vi "n64_generate_grid.vi"(8 "Tare":bool=TRUE, 9 "Row Length":i32=64, 10 "No. Nodes":i32=64, 11 "Sensor Readings (PACKET)":i16[](array[numeric])) -> (0 "Node XYZ List":dbl[][](array[numeric]), 1 "Y (GRID)":dbl[][](array[numeric]), 2 "X (GRID)":dbl[][](array[numeric]), 3 "Z (GRID)":dbl[][](array[numeric]))   [LabVIEW 2016]
uses:
  <vilib>/Math Plots/3D Math Plots/3D Quiver/3D Quiver XCtrl/3D Quiver.xctl
  <vilib>/Math Plots/3D Math Plots/3D Quiver/3D Quiver Datatype/Public/Plot Helper (Matrix).vi
  <vilib>/Math Plots/3D Math Plots/3D Quiver/3D Quiver Datatype/3D Quiver Datatype.lvclass
panel:
  in  "Tab Control":enum32{"16 Node", "64 Node"}(tab)
  in  "Lookup Index n16":i32[](array[numeric])=[0, 1, 2, 3, 4, 5, 6, 7, 8, 9, 10, 11, 12, 13, 14, 15]
  in  "Inv Gain n16":i32[][](array[numeric])=[[1, 1, 1], [1, 1, 1], [1, 1, 1], [1, 1, 1], [1, 1, 1], [1, 1, 1], [1, 1, 1], [1, 1, 1], [1, 1, 1], [1, 1, 1], [1, 1, 1], [1, 1, 1], [1, 1, 1], [1, 1, 1], [1, 1, 1], [1, 1, 1]]
  in  "Lookup Index n64":i32[](array[numeric])=[0, 1, 2, 3, 4, 5, 6, 7, 8, 9, 10, 11, 12, 13, 14, 15, 16, 17, 18, 19, 20, 21, 22, 23, 24, 25, 26, 27, 28, 29, 30, 31, 32, 33, 34, 35, 36, 37, 38, 39, 40, 41, 42, 43, 44, 45, 46, 47, 48, 49, 50, 51, 52, 53, 54, 55, 56, 57, 58, 59, 60, 61, 62, 63]
  in  "Inv Gain n64":i32[][](array[numeric])=[[1, 1, 1], [1, 1, 1], [1, 1, 1], [1, 1, 1], [1, 1, 1], [1, 1, 1], [1, 1, 1], [1, 1, 1], [1, 1, 1], [1, 1, 1], [1, 1, 1], [1, 1, 1], [1, 1, 1], [1, 1, 1], [1, 1, 1], [1, 1, 1], [1, 1, 1], [1, 1, 1], [1, 1, 1], [1, 1, 1], [1, 1, 1], [1, 1, 1], [1, 1, 1], [1, 1, 1], [1, 1, 1], [1, 1, 1], [1, 1, 1], [1, 1, 1], [1, 1, 1], [1, 1, 1], [1, 1, 1], [1, 1, 1], [1, 1, 1], [1, 1, 1], [1, 1, 1], [1, 1, 1], [1, 1, 1], [1, 1, 1], [1, 1, 1], [1, 1, 1], [1, 1, 1], [1, 1, 1], [1, 1, 1], [1, 1, 1], [1, 1, 1], [1, 1, 1], [1, 1, 1], [1, 1, 1], [1, 1, 1], [1, 1, 1], [1, 1, 1], [1, 1, 1], [1, 1, 1], [1, 1, 1], [1, 1, 1], [1, 1, 1], [1, 1, 1], [1, 1, 1], [1, 1, 1], [1, 1, 1], [1, 1, 1], [1, 1, 1], [1, 1, 1], [1, 1, 1]]
  in  "Tare":dbl[][](array[numeric])=[[0.00018775, -0.000174232, 3312.98], [0.000139686, -0.00039953199999999997, 2906.42], [-0.000288384, -0.001229387, 2606.34], [-3.6799e-05, -0.0012016, 3702.6], [0.000266605, -0.001108476, 3847.7999999999997], [0.00038301, -0.000208027, 3472.7], [-0.000177236, -0.000316171, 3651.7799999999997], [-0.00024557699999999997, 0.000544475, 4767.4], [-5.6325e-05, -0.00041305, 4172.08], [8.4112e-05, 0.000956774, 2562.7799999999997], [-0.000261348, 0.001097962, 3675.98], [-0.00014944899999999998, -0.00066839, 4856.94], [-0.000204272, 0.000920726, 4740.78], [-0.000242573, -7.7353e-05, 4009.94], [0.000246328, -0.000138184, 4358.42], [7.51e-06, 0.000451351, 5829.78]]
  out "3D Quiver":refnum<class "3D Plot Datatype.lvclass">[](xcontrol)
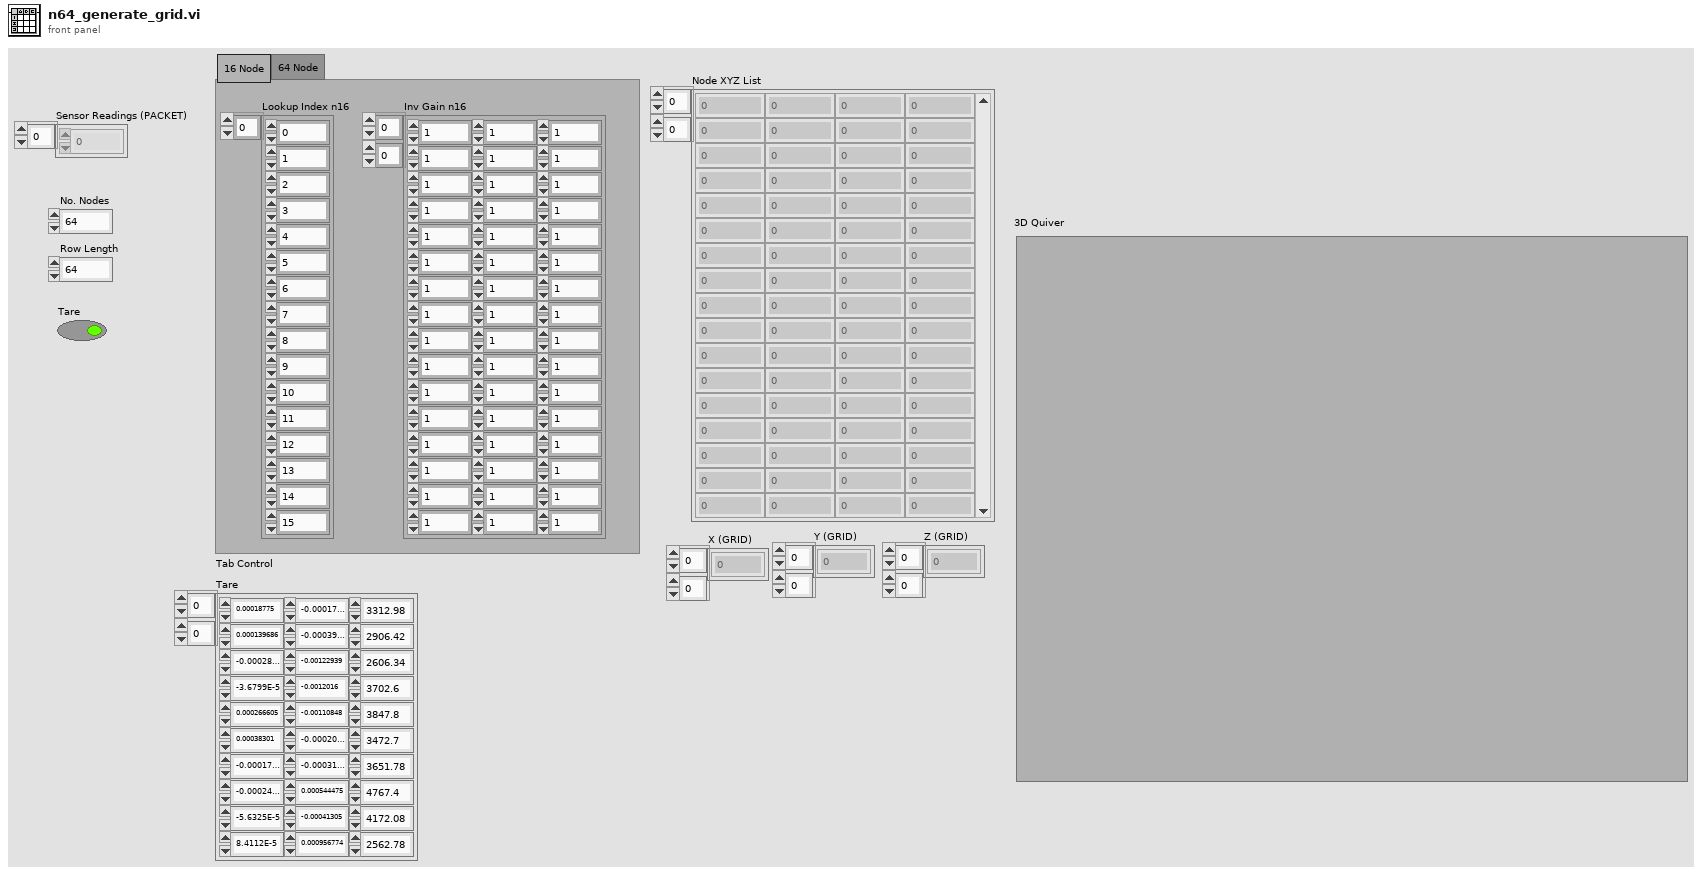
[diagram p1: front panel]
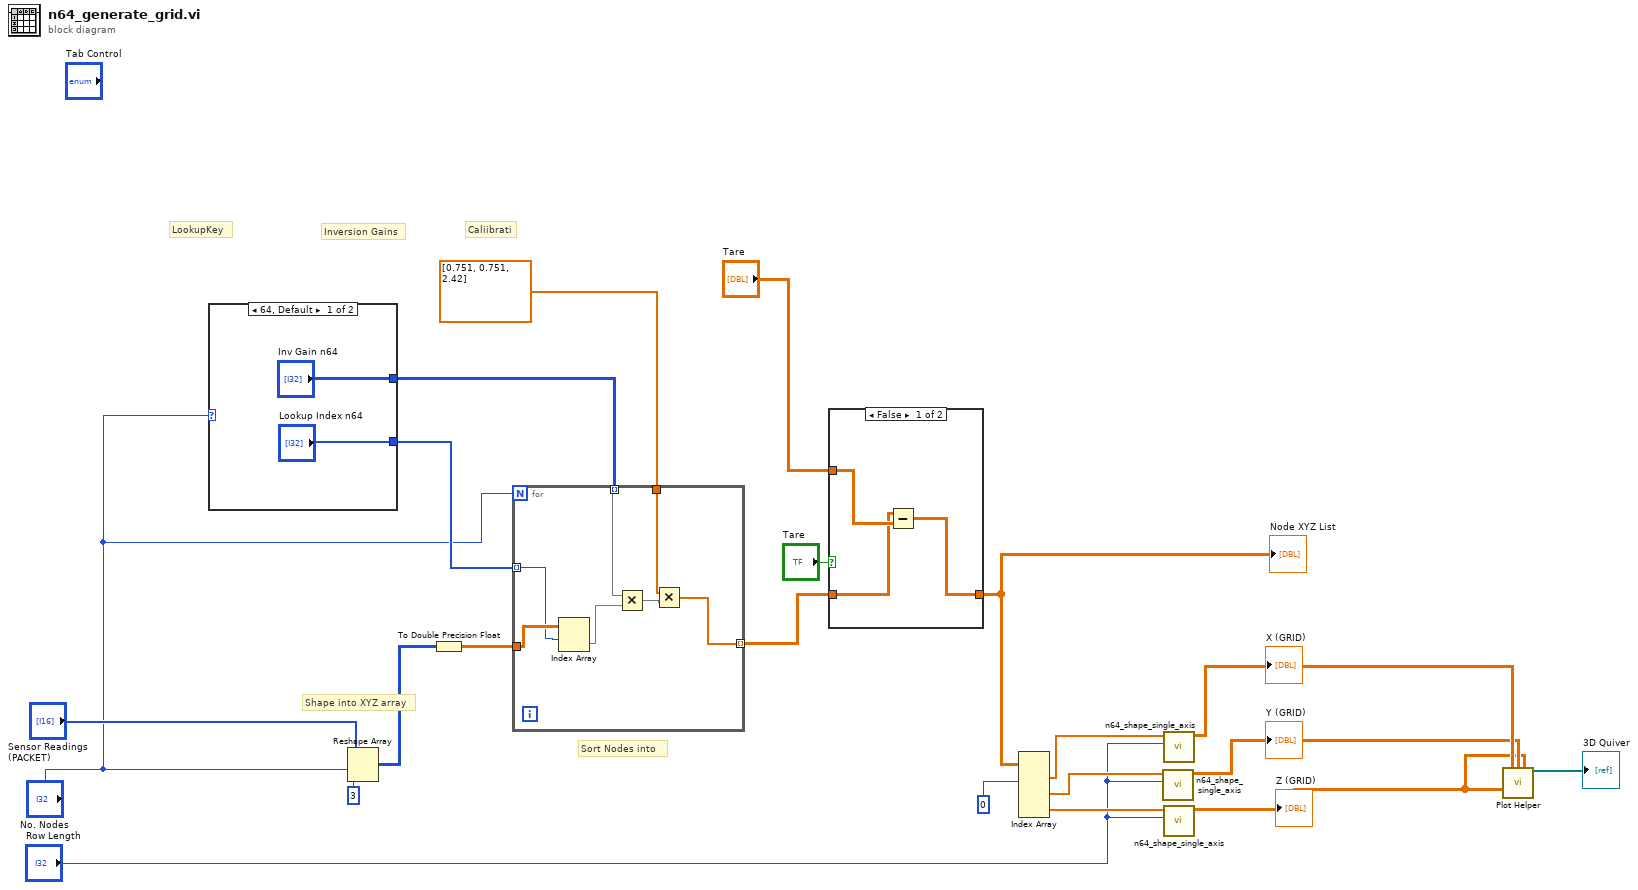
[diagram p0: block diagram]
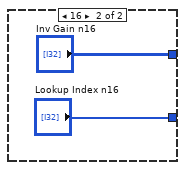
[diagram p2: hidden frame]
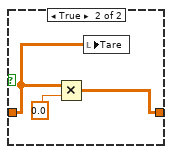
[diagram p3: hidden frame]
diagram:
  # "Caliibrati"
  # "Inversion Gains"
  # "LookupKey"
  # "Sort Nodes into"
  # "Shape into XYZ array"
  n1 = case shown="64, Default" "No. Nodes" {
    tunnel: ["Lookup Index n64" "Lookup Index n16"] -> w14
    tunnel: ["Inv Gain n64" "Inv Gain n16"] -> w12
    frame 64, Default {
    }
    frame 16 {
    }
  }
  n2 = Reshape Array("Sensor Readings (PACKET)", "No. Nodes", 3 ("milliseconds to wait")) -> (w11:i16[][])
  n3 = To Double Precision Float(number=w11) -> (double precision float=w10:dbl[][])
  n4 = for {
    N: "No. Nodes" -> [_]
    tunnel: w10 -> [w32]
    tunnel: w14 -> [w26] mode=indexing
    tunnel: [w27] -> w9 mode=indexing
    tunnel: dbl[] [0.751, 0.751, 2.42] -> [w29]
    tunnel: w12 -> [w31] mode=indexing
    n5 = Index Array(array=w32, index (row)=w26) -> (element=w28:dbl[])  [unwired: 1 in]
    n6 = Multiply(x=w31, y=w28) -> (x*y=w30:dbl[])
    n7 = Multiply(x=w29, y=w30) -> (x*y=w27:dbl[])
  }
  n8 = case shown="False" "Tare" {
    tunnel: w9 -> [w33 w38]
    tunnel: [w35 w36] -> w8
    tunnel: "Tare" -> [w34 _]
    frame False {
      n9 = Subtract(x=w33, y=w34) -> (x-y=w35:dbl[][])
    }
    frame True {
      n10 = Multiply(x=w38, y=0.0 ("milliseconds to wait")) -> (x*y=w36:dbl[][])
      n11 = local write "Tare"(w38) -> ()
    }
  }
  "Node XYZ List" <- w8
  n12 = Index Array(array=w8, index (col) #1=0 ("disabled index (col)")) -> (element #1=w17:dbl[], element #2=w16:dbl[], element #3=w20:dbl[])  [unwired: 5 in]
  n13 = call "n64_shape_single_axis.vi"("Row Length"="Row Length", "Readings (FLAT)"=w16) -> ("Readings (GRID)"=w4:dbl[][])  [unwired: 9 in]
  "Y (GRID)" <- w4
  n14 = call "n64_shape_single_axis.vi"("Row Length"="Row Length", "Readings (FLAT)"=w17) -> ("Readings (GRID)"=w5:dbl[][])  [unwired: 9 in]
  "X (GRID)" <- w5
  n15 = call "n64_shape_single_axis.vi"("Row Length"="Row Length", "Readings (FLAT)"=w20) -> ("Readings (GRID)"=w3:dbl[][])  [unwired: 9 in]
  "Z (GRID)" <- w3
  n16 = call-poly <vilib>:"Plot Helper.vi"("Nx matrix"=w5, "Ny matrix"=w4, "Nz matrix"=w3, "z matrix"=w3) -> ("3D Plot lvclass Array out"=→"3D Quiver":refnum<class "3D Plot Datatype.lvclass">[])  [unwired: 5 in, 6 out]
